vi "0-Do Overlays.vi"(8 "Image Descriptor":T7, 9 "Current Waypoint #":T1, 10 "Waypoints List":T2, 11 "Image in":T6) -> (3 "Image out":T6)   [LabVIEW 2011]
doc: "Overlays waypoints and a boat icon on the image."
uses:
  <vilib>/vision/Image Controls.llb/IMAQ Image.ctl
  0-Image Descriptor.ctl
  2-Think/2 Typedefs/UTM Location.ctl
  0x2-OCU-Think Comm/0x2 Typedefs/Waypoints List.ctl
  0x2-OCU-Think Comm/0x2 Typedefs/ocuWaypoint.ctl
  0x2-OCU-Think Comm/0x2 Typedefs/waypointTypes.ctl
  0x2-OCU-Think Comm/0x2 Typedefs/Current Waypoint.ctl
  2-Think/2 Globals/2 Global.vi
panel:
  out "Boat Outside Img":bool
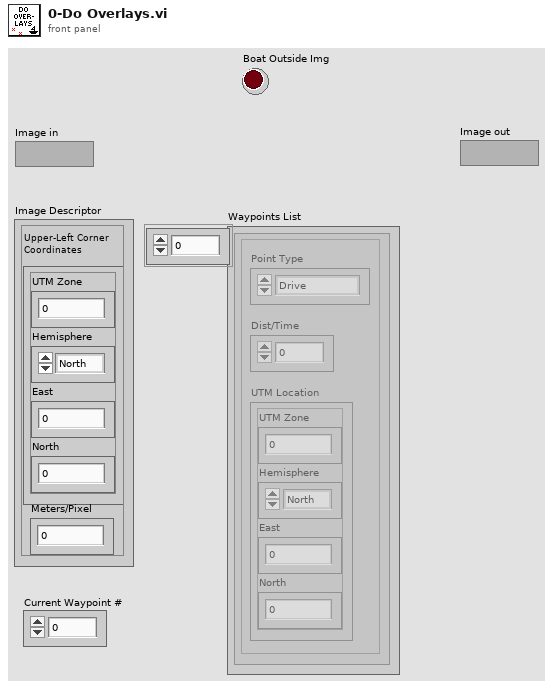
[diagram p1: front panel]
types:
  T1 = typedef "Current Waypoint.ctl" = i32
  T2 = typedef "Waypoints List.ctl" = T3[]
  T3 = typedef "ocuWaypoint.ctl" = cluster{"Point Type":T4, "Dist/Time":dbl, "UTM Location":T5}
  T4 = typedef "waypointTypes.ctl" = enum16{"Drive", "Round Port", "Round Starboard", "Stay"}
  T5 = typedef "UTM Location.ctl" = cluster{"UTM Zone":dbl, "Hemisphere":enum16{"North", "South"}, "East":dbl, "North":dbl}
  T6 = typedef "IMAQ Image.ctl" = refnum<image>
  T7 = typedef "0-Image Descriptor.ctl" = cluster{"Upper-Left Corner Coordinates":T5, "Meters/Pixel":dbl}
  T8 = typedef "Overlay References.ctl" = cluster{"Boat Icon, Unroatated":T6, "Boat Icon, Rotated":T6, "Sail Icon, Unrotated":T6, "Sail Icon, Rotated":T6}
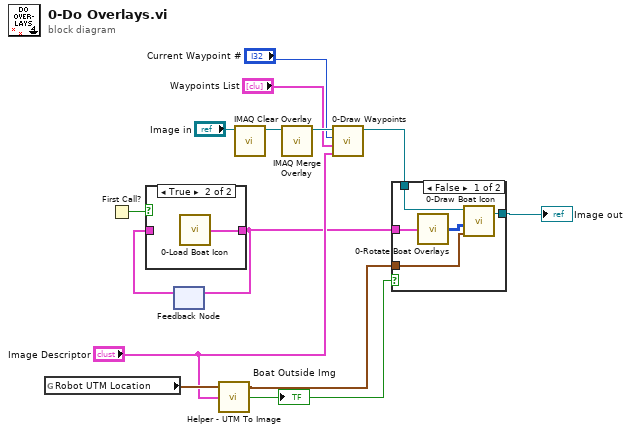
[diagram p0: block diagram]
diagram:
  n1 = global read "2 Global.vi" "Robot UTM Location"() -> (w13:T5)
  n2 = First Call?() -> (First Call?: T/F=w7:bool)
  n3 = feedback #1() -> (w5:T8)  [unwired: 1 in]
  n4 = case shown="True" w7 {
    tunnel: [w15 w16] -> w6
    tunnel: w5 -> [w15 _]
    frame False {
      # "image already\nloaded"
    }
    frame True {
      n5 = call "0-Load Boat Icon.vi"() -> ("Overlay References Out"=w16:T8)  [unwired: 1 in]
    }
  }
  n6 = feedback-in #1(w6) -> ()
  n7 = call "Helper - UTM To Image.vi"("Image Descriptor"="Image Descriptor", "UTM Location"=w13) -> ("Coordinate Outside Image"=w2:bool, "Pixel Coordinates"=w1:cluster{"X":i32, "Y":i32})  [unwired: 1 in, 1 out]
  "Boat Outside Img" <- w2
  n8 = call "IMAQ Clear Overlay"("Image"="Image in") -> ("Image Out"=w14:T6)  [unwired: 2 in, 8 out]
  n9 = call "IMAQ Merge Overlay"("Image Src"=w14) -> ("Image Dst Out"=w10:T6)  [unwired: 4 in, 6 out]
  n10 = call "0-Draw Waypoints.vi"("Image Descriptor"="Image Descriptor", "Waypoints List"="Waypoints List", "Current Waypoint #"="Current Waypoint #", "Image In"=w10) -> ("Image Out"=w11:T6)  [unwired: 2 in, 1 out]
  n11 = case shown="False" w2 {
    tunnel: [w21 w22] -> w12
    tunnel: w11 -> [w20 w22]
    tunnel: w1 -> [w19 _]
    tunnel: w6 -> [w18 _]
    frame False {
      n12 = call "0-Rotate Boat Overlays.vi"("Overlay References In"=w18) -> ("Rotated Boat Icon Bitmap Out"=w17:u32[][])  [unwired: 3 in, 1 out]
      n13 = call "0-Draw Boat Icon.vi"("Position"=w19, "Boat Bitmap"=w17, "Image In"=w20) -> ("Image Out"=w21:T6)  [unwired: 4 out]
    }
    frame True {
      # "don't draw\nif boat\noutside\nimage"
    }
  }
  "Image out" <- w12
